vi "Create Signals Wrapper.vi"   [LabVIEW 2015]
uses:
  <vilib>/LV-Signals/create-xnode/LV-Create-Signals.xnode
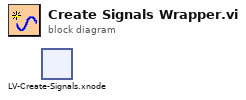
[diagram p0: block diagram]
diagram:
  n1 = xnode "LV-Create-Signals.xnode"() -> ()  [unwired: 2 in, 2 out]
